vi "FOCUS_V42.vi"(9 "X-pixels":sgl=256.0, 11 "Run":bool) -> (0 "Retrace pixels":sgl, 10 "Pixel Clock (Hz)":sgl)   [LabVIEW 2010] (continued)
                    n2566 = local read "stop 2"() -> (w4780:bool)
                    n2567 = Increment(x=w4762) -> (x+1=w4797:i32)
                    "#" <- w4797
                    n2568 = local read "Overlay Images"() -> (w4801:bool)
                    n2569 = Array Subset "Extract DI0"(array=w4763, index=w4788, length=w4790) -> (w4793:u32[])
                    n2570 = Equal?(x=w4797, y=w4776) -> (x = y?=w4778:bool)
                    n2571 = Split Number(x=w4793) -> (hi(x)=w4752:u16[], lo(x)=w4760:u16[])
                    n2572 = case shown="0, Default" w4759 {
                      tunnel: w4752 -> [w4828 w4833 w4838 w4843 w4848 w4853]
                      tunnel: [w4827 w4832 w4835 w4842 w4847 w4850] -> w4757
                      tunnel: [w4825 w4830 w4837 w4840 w4845 w4852] -> w4756
                      tunnel: w4760 -> [w4826 w4831 w4836 w4841 w4846 w4851]
                      tunnel: [w4824 w4829 w4834 w4839 w4844 w4849] -> w4758
                      frame 0, Default {
                        n2573 = Split Number(x=w4828) -> (hi(x)=w4827:u8[], lo(x)=w4825:u8[])
                        n2574 = Split Number(x=w4826) -> (lo(x)=w4824:u8[])  [unwired: 1 out]
                      }
                      frame 1 {
                        n2575 = Split Number(x=w4833) -> (hi(x)=w4832:u8[], lo(x)=w4829:u8[])
                        n2576 = Split Number(x=w4831) -> (lo(x)=w4830:u8[])  [unwired: 1 out]
                      }
                      frame 2 {
                        n2577 = Split Number(x=w4838) -> (hi(x)=w4834:u8[], lo(x)=w4837:u8[])
                        n2578 = Split Number(x=w4836) -> (lo(x)=w4835:u8[])  [unwired: 1 out]
                      }
                      frame 3 {
                        n2579 = Split Number(x=w4843) -> (hi(x)=w4842:u8[], lo(x)=w4840:u8[])
                        n2580 = Split Number(x=w4841) -> (lo(x)=w4839:u8[])  [unwired: 1 out]
                      }
                      frame 4 {
                        n2581 = Split Number(x=w4848) -> (hi(x)=w4847:u8[], lo(x)=w4844:u8[])
                        n2582 = Split Number(x=w4846) -> (lo(x)=w4845:u8[])  [unwired: 1 out]
                      }
                      frame 5 {
                        n2583 = Split Number(x=w4853) -> (hi(x)=w4849:u8[], lo(x)=w4852:u8[])
                        n2584 = Split Number(x=w4851) -> (lo(x)=w4850:u8[])  [unwired: 1 out]
                      }
                    }
                    n2585 = Set File Position(refnum=w4774, from (0:start)=enum16{"start", "end", "current"}."current" ("pos mode (0:2)"), error in=w4773) -> (refnum out=w4749:refnum<file>, error out=w4748:errorcluster)  [unwired: 1 in]
                    n2586 = Compound Arithmetic op=OR(w4778, w4779, w4780, w4782, w4781, w4783, w4784) -> (w4777:bool)
                    n2587 = Tick Count (ms)() -> (millisecond timer value=w4809:u32)
                    n2588 = case shown="1" w4761 {
                      tunnel: w4757 -> [w4856 w4864]
                      tunnel: [w4856 w4863] -> w4755
                      tunnel: w4762 -> [_ w4859]
                      tunnel: w4756 -> [w4855 w4861]
                      tunnel: [w4855 w4860] -> w4754
                      tunnel: w4758 -> [w4854 w4858]
                      tunnel: [w4854 w4857] -> w4753
                      frame 0, Default {
                      }
                      frame 1 {
                        n2589 = local read "Shift"() -> (w4862:sgl)
                        n2590 = call "testoddevenFOCUS.vi"("Numeric"=w4859) -> ("Boolean"=w4865:bool)
                        n2591 = case shown="True" w4865 {
                          tunnel: w4864 -> [w4868 w4895]
                          tunnel: [w4868 w4897] -> w4863
                          tunnel: w4862 -> [_ w4871]
                          tunnel: w4861 -> [w4867 w4883]
                          tunnel: [w4867 w4882] -> w4860
                          tunnel: w4858 -> [w4866 w4870]
                          tunnel: [w4866 w4869] -> w4857
                          frame False {
                          }
                          frame True {
                            n2592 = Round Toward -Infinity(1:w4871) -> (0:w4887:sgl)
                            n2593 = Round Toward -Infinity(1:w4871) -> (0:w4878:sgl)
                            n2594 = Round Toward -Infinity(1:w4871) -> (0:w4902:sgl)
                            n2595 = To Word Integer(number=w4883) -> (16bit integer=w4893:i16[])
                            n2596 = To Word Integer(number=w4870) -> (16bit integer=w4872:i16[])
                            n2597 = To Word Integer(number=w4895) -> (16bit integer=w4894:i16[])
                            n2598 = Array Subset(array=w4893, index=1) -> (w4886:i16[])  [unwired: 1 in]
                            n2599 = Array Subset(array=w4872, index=1) -> (w4879:i16[])  [unwired: 1 in]
                            n2600 = Array Subset(array=w4894, index=1) -> (w4903:i16[])  [unwired: 1 in]
                            n2601 = Subtract(x=w4871, y=w4887) -> (x-y=w4888:sgl)
                            n2602 = Subtract(x=w4871, y=w4878) -> (x-y=w4877:sgl)
                            n2603 = Subtract(x=w4871, y=w4902) -> (x-y=w4901:sgl)
                            n2604 = Subtract(x=w4893, y=w4886) -> (x-y=w4890:i16[])
                            n2605 = Subtract(x=w4872, y=w4879) -> (x-y=w4875:i16[])
                            n2606 = Subtract(x=w4894, y=w4903) -> (x-y=w4899:i16[])
                            n2607 = Build Array (concatenate)(0 ("index"), w4890) -> (w4891:i32[])
                            n2608 = Build Array (concatenate)(0 ("index"), w4875) -> (w4874:i32[])
                            n2609 = Build Array (concatenate)(0 ("index"), w4899) -> (w4898:i32[])
                            n2610 = Multiply(x=w4888, y=w4891) -> (x*y=w4889:sgl[])
                            n2611 = Multiply(x=w4877, y=w4874) -> (x*y=w4876:sgl[])
                            n2612 = Multiply(x=w4901, y=w4898) -> (x*y=w4900:sgl[])
                            n2613 = Add(x=w4893, y=w4889) -> (x+y=w4884:sgl[])
                            n2614 = To Unsigned Byte Integer(number=w4884) -> (unsigned 8bit integer=w4882:u8[])
                            n2615 = Add(x=w4872, y=w4876) -> (x+y=w4881:sgl[])
                            n2616 = To Unsigned Byte Integer(number=w4881) -> (unsigned 8bit integer=w4869:u8[])
                            n2617 = Add(x=w4894, y=w4900) -> (x+y=w4905:sgl[])
                            n2618 = To Unsigned Byte Integer(number=w4905) -> (unsigned 8bit integer=w4897:u8[])
                          }
                        }
                      }
                    }
                    n2619 = case shown="True" w4801 {
                      tunnel: w4755 -> [w4925 w4928]
                      tunnel: [w4925 w4926] -> w4803
                      tunnel: w4754 -> [w4924 w4927]
                      tunnel: [w4924 _] -> w4802
                      frame False {
                      }
                      frame True {
                        n2620 = To Word Integer(number=w4928) -> (16bit integer=w4933:i16[])
                        n2621 = Subtract(x=w4933, y=w4927) -> (x-y=w4934:i16[])
                        n2622 = Add(x=w4933, y=w4927) -> (x+y=w4938:i16[])
                        n2623 = Increment(x=w4938) -> (x+1=w4929:i16[])
                        n2624 = Divide(x=w4934, y=w4929) -> (x/y=w4930:dbl[])
                        n2625 = Absolute Value(x=w4934) -> (abs(x)=w4936:i16[])
                        n2626 = Multiply(x=w4930, y=u8 2) -> (x*y=w4932:dbl[])
                        n2627 = Round To Nearest(number=w4932) -> (nearest integer value=w4945:dbl[])
                        n2628 = Divide(x=w4936, y=2.0) -> (x/y=w4939:dbl[])
                        n2629 = Divide(x=w4938, y=2.0) -> (x/y=w4940:dbl[])
                        n2630 = Add(x=w4939, y=w4940) -> (x+y=w4942:dbl[])
                        n2631 = Divide(x=w4942, y=5.0) -> (x/y=w4943:dbl[])
                        n2632 = Round To Nearest(number=w4943) -> (nearest integer value=w4944:dbl[])
                        n2633 = Multiply(x=5.0 ("y"), y=w4944) -> (x*y=w4946:dbl[])
                        n2634 = Add(x=w4945, y=w4946) -> (x+y=w4947:dbl[])
                        n2635 = Subtract(x=w4947, y=2.0) -> (x-y=w4950:dbl[])
                        n2636 = To Unsigned Byte Integer(number=w4950) -> (unsigned 8bit integer=w4926:u8[])
                      }
                    }
                    n2637 = Subtract(x=w4762, y=w4790) -> (x-y=w4791:sgl)
                    n2638 = Subtract(x=w4809, y=w4808) -> (x-y=w4810:u32)
                    n2639 = local read "Image Update [ms]"() -> (w4792:u32)
                    n2640 = property class="DAQmx Read"(reference=w4770, error in=w4768) -> (reference out=w4769:refnum<k21>, error out=w4767:errorcluster, "Status:Available Samples Per Channel"=w4766:u32)
                    n2641 = Greater Or Equal?(x=w4810, y=w4792) -> (x >= y?=w4811:bool)
                    n2642 = local write "Scan Backlock"(w4766) -> ()
                    n2643 = case shown="True" w4750 {
                      tunnel: w4755 -> [w4820 w4823]
                      tunnel: w4754 -> [w4817 w4822]
                      tunnel: w4753 -> [w4819 _]
                      tunnel: [w4818 w4821] -> w4751
                      frame True {
                        n2644 = Interleave 1D Arrays(w4817, w4820, w4819) -> (w4818:u8[])
                      }
                      frame False {
                        n2645 = Interleave 1D Arrays(w4823, w4822) -> (w4821:u8[])
                      }
                    }
                    n2646 = Write to Binary File(file (use dialog)=w4749, data=w4751, error in=w4748, 5:FALSE ("prepend array or string size? (T)")) -> (refnum out=w4772:refnum<file>, error out=w4771:errorcluster)  [unwired: 2 in, 1 out]
                    n2647 = local read "X-pixels"() -> (w4812:sgl)
                    n2648 = Subtract(x=w4762, y=w4812) -> (x-y=w4804:sgl)
                    n2649 = Replace Array Subset(array=w4816, new element=w4803, index (col)=w4762) -> (w4814:u8[][])  [unwired: 1 in]
                    n2650 = Replace Array Subset(array=w4815, new element=w4802, index (col)=w4762) -> (w4813:u8[][])  [unwired: 1 in]
                    n2651 = Array Subset(array=w4814, index (col)=w4804, length (col)=w4812) -> (w4806:u8[][])  [unwired: 2 in]
                    n2652 = Array Subset(array=w4813, index (col)=w4804, length (col)=w4812) -> (w4805:u8[][])  [unwired: 2 in]
                    n2653 = case shown="True" w4811 {
                      tunnel: [w4951 w4954] -> w4807
                      tunnel: w4808 -> [w4951 _]
                      tunnel: w4806 -> [_ w4953]
                      tunnel: w4805 -> [_ w4952]
                      frame False {
                      }
                      frame True {
                        n2654 = local write "Image 2"(w4952) -> ()
                        n2655 = local write "Image 1"(w4953) -> ()
                        n2656 = Tick Count (ms)() -> (millisecond timer value=w4954:u32)
                      }
                    }
                  }
                  n2657 = Close File(refnum=w4698, error in=w4699) -> ()  [unwired: 2 out]
                  n2658 = flat-sequence {
                    tunnel: w4731 -> [w4745]
                    tunnel: [w4745] -> w4730
                    frame #0 {
                      n2659 = Tick Count (ms)() -> (millisecond timer value=w4746:u32)
                      n2660 = local write "stop"(w4746) -> ()
                    }
                  }
                }
                frame 3 {
                  w5004 = 0.0 ("X Scale.Range:Minimum")
                  w5017 = 0.0 ("x offset")
                  w5018 = 1.0 ("x offset")
                  w5006 = TRUE ("Visible")
                  # "User-defined line"
                  n2661 = property on="Property Node" class="VI"() -> ("VI Path"=w4972:path)  [unwired: 2 in, 2 out]
                  n2662 = flat-sequence {
                    tunnel: w5011 -> [w5033]
                    tunnel: [w5033] -> w5010
                    frame #0 {
                      n2663 = Tick Count (ms)() -> (millisecond timer value=w5034:u32)
                      n2664 = local write "start"(w5034) -> ()
                    }
                  }
                  n2665 = Greater Or Equal?(x=w4960, y=u16 3) -> (x >= y?=w4958:bool)
                  n2666 = Strip Path(path=w4972) -> (stripped path=w4971:path)  [unwired: 1 out]
                  n2667 = Tick Count (ms)() -> (millisecond timer value=w5024:u32)
                  n2668 = Bundle("x offset"=w5018, "x offset"=w5018, "x offset"=w5017, "x offset"=w5017) -> (w5016:T33)  [unwired: 1 in]
                  n2669 = Build Path(base path=w4971, name or relative path="FreeLine.tmp") -> (appended path=w4970:path)
                  n2670 = Unbundle By Name(w4986) -> ("status"=w4985:bool)
                  n2671 = call <vilib>:"Open_Create_Replace File.vi"("advisory dialog? (display:T)"=FALSE, "function (open:0)"=T8."create or replace", "file path"=w4970) -> ("error out"=w4964:errorcluster, "refnum"=w4966:refnum<file>)  [unwired: 5 in, 2 out]
                  n2672 = Set File Position(refnum=w4966, from (0:start)=enum16{"start", "end", "current"}."start" ("pos mode (rel. to end:1)"), error in=w4964) -> (refnum out=w4957:refnum<file>, error out=w4956:errorcluster)  [unwired: 1 in]
                  n2673 = Write to Binary File(file (use dialog)=w4957, data=w4962, error in=w4956, 5:FALSE ("prepend array or string size? (T)")) -> (refnum out=w4965:refnum<file>, error out=w4963:errorcluster)  [unwired: 2 in, 1 out]
                  n2674 = while {
                    tunnel: [w5054] -> w5025
                    tunnel: [w5055] -> w5009
                    tunnel: w5026 -> [w5100]
                    tunnel: w5010 -> [w5099]
                    shift-right: [w5115] -> w4978
                    shift-left: w5027 -> [w5141]
                    tunnel: w4988 -> [w5097]
                    shift-right: [w5116] -> w4977
                    shift-left: w5027 -> [w5140]
                    shift-right: [w5134] -> _
                    shift-left: w5024 -> [w5135]
                    tunnel: w5022 -> [w5126]
                    tunnel: w5021 -> [w5090]
                    tunnel: [w5125] -> w5020
                    tunnel: [w5124] -> w5019
                    shift-right: [w5121] -> _
                    shift-left: w5016 -> [w5128]
                    tunnel: w5015 -> [w5103]
                    tunnel: w5014 -> [w5091]
                    tunnel: [w5102] -> w5013
                    tunnel: [w5101] -> w5012
                    shift-right: [w5106] -> w4968
                    shift-left: w5002 -> [w5108]
                    tunnel: w4992 -> [w5104]
                    tunnel: w4991 -> [w5082]
                    tunnel: [w5104] -> w4990
                    tunnel: [w5082] -> w4989
                    tunnel: [w5094] -> w4987
                    tunnel: w4985 -> [w5089]
                    shift-right: [w5058] -> w4976
                    shift-left: w4965 -> [w5061]
                    shift-right: [w5059] -> w4975
                    shift-left: w4963 -> [w5060]
                    tunnel: w4961 -> [w5052]
                    tunnel: w4960 -> [w5044]
                    tunnel: w4958 -> [w5038]
                    i -> [w5093]
                    stop <- w5080 stop-if-true
                    # "DIO Read reads one\nline of data at a time"
                    n2675 = Equal To 0?(x=w5093) -> (x = 0?=w5112:bool)
                    n2676 = local read "End experiment"() -> (w5087:bool)
                    n2677 = case shown="True" w5112 {
                      tunnel: w5097 -> [w5207 w5210]
                      tunnel: [w5207 w5209] -> w5049
                      tunnel: w5052 -> [_ w5208]
                      tunnel: [sgl 0.0 w5208] -> w5048
                      frame False {
                      }
                      frame True {
                        n2678 = Add(x=w5210, y=w5208) -> (x+y=w5209:sgl)
                      }
                    }
                    n2679 = call-poly <vilib>:"DAQmx Read (Digital 1D U32 1Chan NSamp).vi"("task/channels in"=w5100, "number of samples per channel"=w5049, "error in"=w5099) -> ("task out"=w5057:refnum<k21>, "data"=w5051:u32[], "error out"=w5056:errorcluster)  [unwired: 10 in]
                    n2680 = Increment(x=w5093) -> (x+1=w5105:i32)
                    "#" <- w5105
                    n2681 = call-poly <vilib>:"DAQmx Read (Analog 2D DBL NChan NSamp).vi"("task/channels in"=w5103, "number of samples per channel"=w5049, "error in"=w5091) -> ("task out"=w5102:refnum<k21>, "data"=w5047:dbl[][], "error out"=w5101:errorcluster)  [unwired: 10 in]
                    n2682 = Unbundle By Name(w5091) -> ("status"=w5081:bool)
                    n2683 = local read "stop 2"() -> (w5088:bool)
                    n2684 = local read "Overlay Images"() -> (w5109:bool)
                    n2685 = Array Subset(array=w5047, index (col)=w5048) -> (w5046:dbl[][])  [unwired: 3 in]
                    n2686 = Unbundle By Name(w5090) -> ("status"=w5083:bool)
                    n2687 = Equal?(x=w5105, y="Y-lines FreeLine") -> (x = y?=w5086:bool)
                    n2688 = Transpose 2D Array(2D array=w5046) -> (transposed array=w5098:dbl[][])
                    n2689 = Unbundle By Name(w5056) -> ("status"=w5084:bool)
                    n2690 = Array Subset "Extract DI0"(array=w5051, index=w5048) -> (w5050:u32[])  [unwired: 1 in]
                    n2691 = Unbundle By Name(w5082) -> ("status"=w5085:bool)
                    n2692 = Split Number(x=w5050) -> (hi(x)=w5040:u16[], lo(x)=w5045:u16[])
                    n2693 = Build Array (concatenate)(w5108, w5098) -> (w5107:dbl[][])
                    n2694 = Index Array(array=w5098, index (col)=0 ("disabled index (col)")) -> (element=w5118:dbl[])  [unwired: 1 in]
                    n2695 = Bundle("x offset"="x offset", "x scale"="x scale", "y offset"="y offset", "y scale"="y scale") -> (w5121:T34)  [unwired: 1 in]
                    n2696 = Array Subset(array=w5107, index (row)=w5097) -> (w5106:dbl[][])  [unwired: 3 in]
                    n2697 = Index Array(array=w5098, index (col)=1 ("disabled index (col)")) -> (element=w5117:dbl[])  [unwired: 1 in]
                    n2698 = Tick Count (ms)() -> (millisecond timer value=w5136:u32)
                    n2699 = Not Equal?(x=w5128, y=w5121) -> (x != y?=w5127:bool)
                    n2700 = Compound Arithmetic op=OR(w5081, w5083, w5084, w5085, w5086, w5087, w5088, w5089) -> (w5080:bool)
                    n2701 = case shown="True" w5127 {
                      tunnel: w5126 -> [w5212 w5217]
                      tunnel: w5090 -> [w5211 w5214]
                      tunnel: [w5212 w5215] -> w5125
                      tunnel: [w5211 w5213] -> w5124
                      tunnel: w5121 -> [_ w5219]
                      frame False {
                      }
                      frame True {
                        n2702 = local read "ScanLineFreeLine"() -> (w5218:sgl[][])
                        n2703 = call "ScaleudlFOCUS.vi"("Cluster"=w5219, "ScanLineUDL"=w5218) -> ("ScanLineUDLnew"=w5216:dbl[][])
                        n2704 = call-poly <vilib>:"DAQmx Write (Analog 2D DBL NChan NSamp).vi"("task/channels in"=w5217, "data"=w5216, "error in"=w5214) -> ("task out"=w5215:refnum<k21>, "error out"=w5213:errorcluster)  [unwired: 10 in, 1 out]
                      }
                    }
                    n2705 = case shown="0, Default" w5044 {
                      tunnel: w5040 -> [w5153 w5158 w5163 w5168 w5173 w5178]
                      tunnel: [w5152 w5157 w5160 w5167 w5172 w5175] -> w5041
                      tunnel: [w5150 w5155 w5162 w5165 w5170 w5177] -> w5042
                      tunnel: w5045 -> [w5151 w5156 w5161 w5166 w5171 w5176]
                      tunnel: [w5149 w5154 w5159 w5164 w5169 w5174] -> w5043
                      frame 0, Default {
                        n2706 = Split Number(x=w5153) -> (hi(x)=w5152:u8[], lo(x)=w5150:u8[])
                        n2707 = Split Number(x=w5151) -> (lo(x)=w5149:u8[])  [unwired: 1 out]
                      }
                      frame 1 {
                        n2708 = Split Number(x=w5158) -> (hi(x)=w5157:u8[], lo(x)=w5154:u8[])
                        n2709 = Split Number(x=w5156) -> (lo(x)=w5155:u8[])  [unwired: 1 out]
                      }
                      frame 2 {
                        n2710 = Split Number(x=w5163) -> (hi(x)=w5159:u8[], lo(x)=w5162:u8[])
                        n2711 = Split Number(x=w5161) -> (lo(x)=w5160:u8[])  [unwired: 1 out]
                      }
                      frame 3 {
                        n2712 = Split Number(x=w5168) -> (hi(x)=w5167:u8[], lo(x)=w5165:u8[])
                        n2713 = Split Number(x=w5166) -> (lo(x)=w5164:u8[])  [unwired: 1 out]
                      }
                      frame 4 {
                        n2714 = Split Number(x=w5173) -> (hi(x)=w5172:u8[], lo(x)=w5169:u8[])
                        n2715 = Split Number(x=w5171) -> (lo(x)=w5170:u8[])  [unwired: 1 out]
                      }
                      frame 5 {
                        n2716 = Split Number(x=w5178) -> (hi(x)=w5174:u8[], lo(x)=w5177:u8[])
                        n2717 = Split Number(x=w5176) -> (lo(x)=w5175:u8[])  [unwired: 1 out]
                      }
                    }
                    n2718 = case shown="True" w5109 {
                      tunnel: w5041 -> [w5180 w5183]
                      tunnel: [w5180 w5181] -> w5111
                      tunnel: w5042 -> [w5179 w5182]
                      tunnel: [w5179 _] -> w5110
                      frame False {
                      }
                      frame True {
                        n2719 = To Word Integer(number=w5183) -> (16bit integer=w5188:i16[])
                        n2720 = Subtract(x=w5188, y=w5182) -> (x-y=w5189:i16[])
                        n2721 = Add(x=w5188, y=w5182) -> (x+y=w5193:i16[])
                        n2722 = Increment(x=w5193) -> (x+1=w5184:i16[])
                        n2723 = Divide(x=w5189, y=w5184) -> (x/y=w5185:dbl[])
                        n2724 = Absolute Value(x=w5189) -> (abs(x)=w5191:i16[])
                        n2725 = Multiply(x=w5185, y=u8 2) -> (x*y=w5187:dbl[])
                        n2726 = Round To Nearest(number=w5187) -> (nearest integer value=w5200:dbl[])
                        n2727 = Divide(x=w5191, y=2.0) -> (x/y=w5194:dbl[])
                        n2728 = Divide(x=w5193, y=2.0) -> (x/y=w5195:dbl[])
                        n2729 = Add(x=w5194, y=w5195) -> (x+y=w5197:dbl[])
                        n2730 = Divide(x=w5197, y=5.0) -> (x/y=w5198:dbl[])
                        n2731 = Round To Nearest(number=w5198) -> (nearest integer value=w5199:dbl[])
                        n2732 = Multiply(x=5.0 ("y"), y=w5199) -> (x*y=w5201:dbl[])
                        n2733 = Add(x=w5200, y=w5201) -> (x+y=w5202:dbl[])
                        n2734 = Subtract(x=w5202, y=2.0) -> (x-y=w5205:dbl[])
                        n2735 = To Unsigned Byte Integer(number=w5205) -> (unsigned 8bit integer=w5181:u8[])
                      }
                    }
                    n2736 = Subtract(x=w5136, y=w5135) -> (x-y=w5137:u32)
                    n2737 = local read "Image Update [ms]"() -> (w5096:u32)
                    n2738 = property class="DAQmx Read"(reference=w5057, error in=w5056) -> (reference out=w5054:refnum<k21>, error out=w5055:errorcluster, "Status:Available Samples Per Channel"=w5053:u32)
                    n2739 = Multiply(x="x scale", y=w5118) -> (x*y=w5132:dbl[])
                    n2740 = Greater Or Equal?(x=w5137, y=w5096) -> (x >= y?=w5138:bool)
                    n2741 = Multiply(x=w5117, y="y scale") -> (x*y=w5131:dbl[])
                    n2742 = case shown="True" w5038 {
                      tunnel: w5041 -> [w5145 w5148]
                      tunnel: w5042 -> [w5142 w5147]
                      tunnel: w5043 -> [w5144 _]
                      tunnel: [w5143 w5146] -> w5039
                      frame True {
                        n2743 = Interleave 1D Arrays(w5142, w5145, w5144) -> (w5143:u8[])
                      }
                      frame False {
                        n2744 = Interleave 1D Arrays(w5148, w5147) -> (w5146:u8[])
                      }
                    }
                    n2745 = Add(x="x offset", y=w5132) -> (x+y=w5064:dbl[])
                    n2746 = Add(x=w5131, y="y offset") -> (x+y=w5066:dbl[])
                    n2747 = local write "Scan Backlock"(w5053) -> ()
                    n2748 = local read "y jog"() -> (w5067:sgl)
                    n2749 = local read "x jog"() -> (w5068:sgl)
                    n2750 = Subtract(x=w5066, y=w5067) -> (x-y=w5065:dbl[])
                    n2751 = Subtract(x=w5064, y=w5068) -> (x-y=w5063:dbl[])
                    n2752 = local read "Zoom"() -> (w5069:sgl)
                    n2753 = local read "X-pixels FreeLine"() -> (w5095:sgl)
                    n2754 = Replace Array Subset(array=w5141, new element=w5111, index (col)=w5093) -> (w5115:u8[][])  [unwired: 1 in]
                    n2755 = Replace Array Subset(array=w5140, new element=w5110, index (col)=w5093) -> (w5116:u8[][])  [unwired: 1 in]
                    n2756 = Multiply(x=w5065, y=w5069) -> (x*y=w5071:dbl[])
                    n2757 = Multiply(x=w5063, y=w5069) -> (x*y=w5070:dbl[])
                    n2758 = Subtract(x=w5093, y=w5095) -> (x-y=w5139:sgl)
                    n2759 = Set File Position(refnum=w5061, from (0:start)=enum16{"start", "end", "current"}."current" ("pos mode (0:2)"), error in=w5060) -> (refnum out=w5037:refnum<file>, error out=w5036:errorcluster)  [unwired: 1 in]
                    n2760 = Write to Binary File(file (use dialog)=w5037, data=w5039, error in=w5036, 5:FALSE ("prepend array or string size? (T)")) -> (refnum out=w5058:refnum<file>, error out=w5059:errorcluster)  [unwired: 2 in, 1 out]
                    n2761 = Array Subset(array=w5115, index (col)=w5139, length (col)=w5095) -> (w5114:u8[][])  [unwired: 2 in]
                    n2762 = Multiply(x=sgl -2.7 ("X Factor"), y=w5071) -> (x*y=w5077:dbl[])
                    n2763 = Multiply(x=sgl -2.7 ("X Factor"), y=w5070) -> (x*y=w5073:dbl[])
                    n2764 = Subtract(x=w5093, y=w5095) -> (x-y=w5094:sgl)
                    n2765 = Array Subset(array=w5116, index (col)=w5139, length (col)=w5095) -> (w5113:u8[][])  [unwired: 2 in]
                    n2766 = Add(x=sgl -0.005 ("X Offset"), y=w5077) -> (x+y=w5076:dbl[])
                    n2767 = Add(x=sgl -0.025 ("X Offset"), y=w5073) -> (x+y=w5072:dbl[])
                    n2768 = Bundle(w5072, w5076) -> (w5133:cluster{dbl[], dbl[]})  [unwired: 1 in]
                    n2769 = case shown="True" w5138 {
                      tunnel: [w5220 w5224] -> w5134
                      tunnel: w5135 -> [w5220 _]
                      tunnel: w5133 -> [_ w5223]
                      tunnel: w5114 -> [_ w5222]
                      tunnel: w5113 -> [_ w5221]
                      frame False {
                      }
                      frame True {
                        n2770 = local write "XY Graph 3"(w5223) -> ()
                        n2771 = local write "XY Graph 4"(w5223) -> ()
                        n2772 = local write "Image 4"(w5221) -> ()
                        n2773 = local write "Image 3"(w5222) -> ()
                        n2774 = Tick Count (ms)() -> (millisecond timer value=w5224:u32)
                      }
                    }
                  }
                  n2775 = local read "X-pixels FreeLine"() -> (w5007:sgl)
                  n2776 = property on="Image 2" class="IntGraph (strict)"() -> ("Color Table"=w5005:u32[])  [unwired: 2 in, 2 out]
                  n2777 = Decrement(x=w5007) -> (x-1=w5003:sgl)
                  n2778 = property on="Image 3" class="IntGraph (strict)"("X Scale.Range:Minimum"=w5004, "X Scale.Range:Maximum"=w5003, "Y Scale.Range:Minimum"=w5004, "Y Scale.Range:Maximum"=w5003, "Visible"=w5006, "Color Table"=w5005) -> ()  [unwired: 2 in, 2 out]
                  n2779 = property on="Image 4" class="IntGraph (strict)"("X Scale.Range:Minimum"=w5004, "X Scale.Range:Maximum"=w5003, "Y Scale.Range:Minimum"=w5004, "Y Scale.Range:Maximum"=w5003, "Visible"=w5006, "Color Table"=w5005) -> ()  [unwired: 2 in, 2 out]
                  n2780 = property on="Histogram1" class="XYGraph (strict)"("X Scale.Range:Minimum"=w5004, "X Scale.Range:Maximum"=w5003) -> ()  [unwired: 2 in, 2 out]
                  n2781 = property on="Histogram2" class="XYGraph (strict)"("X Scale.Range:Minimum"=w5004, "X Scale.Range:Maximum"=w5003) -> ()  [unwired: 2 in, 2 out]
                  n2782 = Close File(refnum=w4976, error in=w4975) -> ()  [unwired: 2 out]
                  n2783 = Array Subset(array=w4968, index (col)=0 ("index"), length (col)=3 ("length")) -> (w4993:dbl[][])  [unwired: 2 in]
                  n2784 = Index Array(array=w4993, index (col)=0 ("disabled index (col)")) -> (element=w5000:dbl[])  [unwired: 1 in]
                  n2785 = Array Size(array=w5000) -> (size(s)=w4999:i32)
                  n2786 = Multiply(x=w4999, y=3) -> (x*y=w4997:i32)
                  n2787 = Reshape Array(w4993, w4997) -> (→"Positions":dbl[])
                  n2788 = flat-sequence {
                    tunnel: [w5031] -> w5008
                    tunnel: w5009 -> [w5031]
                    frame #0 {
                      n2789 = Tick Count (ms)() -> (millisecond timer value=w5032:u32)
                      n2790 = local write "stop"(w5032) -> ()
                    }
                  }
                }
                frame 4 {
                  # "Iinner while loop runs for n loops, where n = number of averages.\nAll data acquired in this loop enters the average.\nThe z-step is activated each time this loop completes..\nThe outer while loop iterates m times, where m is total number of frames.\nControls are reset after the outer while loop completes.\nThe shutter is closed before and opened after each z-step."
                  # "Frame scan piezo"
                  n2791 = local read "z-step (um)"() -> (w5230:sgl)
                  n2792 = flat-sequence {
                    tunnel: w5287 -> [w5304]
                    tunnel: [w5304] -> w5286
                    frame #0 {
                      n2793 = Tick Count (ms)() -> (millisecond timer value=w5305:u32)
                      n2794 = local write "start"(w5305) -> ()
                    }
                  }
                  n2795 = local read "Number of frames"() -> (w5288:sgl)
                  n2796 = Unbundle By Name(w5257) -> ("status"=w5256:bool)
                  n2797 = local read "z-step (um)"() -> (w5295:sgl)
                  n2798 = property on="Property Node" class="VI"() -> ("VI Path"=w5244:path)  [unwired: 2 in, 2 out]
                  n2799 = Initialize Array(u8 0 ("element"), w5271, w5272) -> (w5284:u8[][])
                  n2800 = Equal To 0?(x=w5230) -> (x = 0?=w5229:bool)
                  n2801 = Initialize Array(0.0 ("element"), 0 ("dimension size")) -> (w5294:dbl[])
                  n2802 = Strip Path(path=w5244) -> (stripped path=w5243:path)  [unwired: 1 out]
                  n2803 = while {
                    tunnel: w5295 -> [w5316]
                    shift-right: [w5314] -> w5290
                    shift-left: w5294 -> [w5315]
                    tunnel: w5288 -> [w5308]
                    i -> [w5307]
                    stop <- w5309 stop-if-true
                    n2804 = Multiply(x=w5316, y=w5307) -> (x*y=w5312:sgl)
                    n2805 = Increment(x=w5307) -> (x+1=w5306:i32)
                    n2806 = Build Array (concatenate)(w5315, w5312) -> (w5314:dbl[])
                    n2807 = Greater Or Equal?(x=w5312, y=400.0) -> (x >= y?=w5310:bool)
                    n2808 = Greater Or Equal?(x=w5306, y=w5308) -> (x >= y?=w5311:bool)
                    n2809 = Or(x=w5310, y=w5311) -> (x .or. y?=w5309:bool)
                  }
                  n2810 = Build Path(base path=w5243, name or relative path="Stack.tmp") -> (appended path=w5242:path)
                  n2811 = call <vilib>:"Open_Create_Replace File.vi"("advisory dialog? (display:T)"=FALSE, "function (open:0)"=T8."create or replace", "file path"=w5242) -> ("error out"=w5235:errorcluster, "refnum"=w5237:refnum<file>)  [unwired: 5 in, 2 out]
                  n2812 = Divide(x=w5290, y=40.0) -> (x/y=w5268:dbl[])
                  n2813 = Set File Position(refnum=w5237, from (0:start)=enum16{"start", "end", "current"}."start" ("pos mode (rel. to end:1)"), error in=w5235) -> (refnum out=w5227:refnum<file>, error out=w5226:errorcluster)  [unwired: 1 in]
                  n2814 = Write to Binary File(file (use dialog)=w5227, data=w5233, error in=w5226, 5:FALSE ("prepend array or string size? (T)")) -> (refnum out=w5236:refnum<file>, error out=w5234:errorcluster)  [unwired: 2 in, 1 out]
                  n2815 = Array Subset(array=w5268, index=1) -> (w5267:dbl[])  [unwired: 1 in]
                  n2816 = local read "IntensityAutomatic"() -> (w5252:bool)
                  n2817 = local read "Intensity"() -> (w5254:sgl)
                  n2818 = while {
                    tunnel: [w5392] -> w5266
                    tunnel: [w5391] -> w5265
                    tunnel: w5300 -> [w5390]
                    tunnel: w5286 -> [w5349]
                    tunnel: w5299 -> [w5325]
                    tunnel: w5289 -> [w5389]
                    tunnel: w5267 -> [w5360] mode=indexing
                    tunnel: w5268 -> [w5388]
                    shift-right: [w5386] -> w5250
                    shift-left: w5284 -> [w5387]
                    shift-right: [w5384] -> w5251
                    shift-left: w5284 -> [w5385]
                    tunnel: w5280 -> [w5383]
                    tunnel: w5279 -> [w5352]
                    tunnel: [w5382] -> w5277
                    tunnel: [w5381] -> w5278
                    tunnel: w5276 -> [w5366]
                    tunnel: w5275 -> [w5365]
                    tunnel: [w5371] -> w5274
                    tunnel: [w5370] -> w5273
                    tunnel: [w5356] -> w5270
                    tunnel: w5260 -> [w5364]
                    tunnel: [w5357] -> w5261
                    tunnel: w5254 -> [w5359]
                    tunnel: w5259 -> [w5355]
                    tunnel: [w5353] -> w5258
                    tunnel: w5256 -> [w5347]
                    tunnel: [w5341] -> w5253
                    tunnel: w5252 -> [w5340]
                    shift-right: [w5336] -> w5240
                    shift-left: w5236 -> [w5338]
                    shift-right: [w5335] -> w5239
                    shift-left: w5234 -> [w5337]
                    tunnel: w5232 -> [w5331]
                    tunnel: w5231 -> [w5322]
                    tunnel: w5229 -> [w5328]
                    tunnel: w5228 -> [w5321]
                    i -> [w5353]
                    stop <- w5327 stop-if-true
                    n2819 = Equal To 0?(x=w5353) -> (x = 0?=w5329:bool)
                    n2820 = Or(x=w5329, y=w5328) -> (x .or. y?=w5330:bool)
                    n2821 = case shown="False" w5330 {
                      tunnel: w5366 -> [w5468 w5477]
                      tunnel: [w5461 w5477] -> w5361
                      tunnel: w5365 -> [w5467 w5478]
                      tunnel: [w5460 w5478] -> w5351
                      tunnel: w5355 -> [w5465 w5475]
                      tunnel: w5364 -> [w5464 w5476]
                      tunnel: [w5459 w5476] -> w5350
                      tunnel: [w5458 w5475] -> w5363
                      frame False {
                        w5466 = TRUE ("data")
                        n2822 = local write "Shutter open"(w5466) -> ()
                        n2823 = call-poly <vilib>:"DAQmx Write (Digital Bool 1Line 1Point).vi"("task/channels in"=w5468, "data"=w5466, "error in"=w5467) -> ("task out"=w5463:refnum<k21>, "error out"=w5462:errorcluster)  [unwired: 10 in, 1 out]
                        n2824 = flat-sequence {
                          tunnel: w5465 -> [w5474]
                          tunnel: w5464 -> [w5473]
                          tunnel: w5463 -> [w5472]
                          tunnel: [w5472] -> w5461
                          tunnel: [w5471] -> w5460
                          tunnel: w5462 -> [w5471]
                          tunnel: [w5470] -> w5459
                          tunnel: [w5469] -> w5458
                          frame #0 {
                            n2825 = call <vilib>:"DAQmx Start Task.vi"("task/channels in"=w5474, "error in"=w5473) -> ("task out"=w5469:refnum<k21>, "error out"=w5470:errorcluster)  [unwired: 12 in]
                          }
                        }
                      }
                      frame True {
                      }
                    }
                    n2826 = Greater Or Equal?(x=w5321, y=u16 3) -> (x >= y?=w5320:bool)
                    n2827 = local read "Number of frames"() -> (w5354:sgl)
                    n2828 = Tick Count (ms)() -> (millisecond timer value=w5373:u32)
                    n2829 = Array Size(array=w5388) -> (size(s)=w5376:i32)
                    n2830 = Unbundle By Name(w5352) -> ("status"=w5348:bool)
                    n2831 = Increment(x=w5353) -> (x+1=w5372:i32)
                    n2832 = Equal?(x=w5354, y=w5372) -> (x = y?=w5374:bool)
                    n2833 = Equal?(x=w5372, y=w5376) -> (x = y?=w5375:bool)
                    n2834 = Compound Arithmetic op=OR(w5348, w5347) -> (w5345:bool)
                    n2835 = while {
                      tunnel: [w5509] -> w5392
                      tunnel: [w5511] -> w5391
                      tunnel: w5390 -> [w5558]
                      tunnel: w5349 -> [w5557]
                      shift-right: [w5544] -> w5334
                      shift-left: w5325 -> [w5545]
                      tunnel: w5389 -> [w5528]
                      shift-right: [w5540] -> w5333
                      shift-left: w5325 -> [w5543]
                      tunnel: [w5516] -> w5344
                      tunnel: [w5517] -> w5343
                      shift-right: [w5561] -> _
                      shift-left: w5373 -> [w5562]
                      tunnel: [w5532] -> w5369
                      tunnel: w5361 -> [w5532]
                      tunnel: [w5522] -> w5367
                      tunnel: w5351 -> [w5522]
                      tunnel: [w5531] -> w5358
                      tunnel: w5363 -> [w5531]
                      tunnel: [w5523] -> w5362
                      tunnel: w5350 -> [w5523]
                      tunnel: w5345 -> [w5515]
                      tunnel: [w5513] -> w5342
                      tunnel: w5331 -> [w5507]
                      tunnel: w5322 -> [w5496]
                      tunnel: w5329 -> [w5503]
                      shift-right: [w5482] -> w5324
                      shift-left: w5325 -> [w5484]
                      tunnel: w5321 -> [w5481]
                      i -> [w5495]
                      stop <- w5514 stop-if-true
                      # "DIO Read reads one\nline of data at a time"
                      n2836 = local read "z-step (um)"() -> (w5505:sgl)
                      n2837 = local read "Scan Cut-Off (either end)"() -> (w5559:sgl)
                      n2838 = local read "End experiment"() -> (w5517:bool)
                      n2839 = Equal To 0?(x=w5495) -> (x = 0?=w5504:bool)
                      n2840 = Equal To 0?(x=w5505) -> (x = 0?=w5506:bool)
                      n2841 = local read "Overlay Images"() -> (w5560:bool)
                      n2842 = Unbundle By Name(w5523) -> ("status"=w5520:bool)
                      n2843 = Unbundle By Name(w5522) -> ("status"=w5519:bool)
                      n2844 = local read "X-pixels"() -> (w5556:sgl)
                      n2845 = local read "Cusp Delay"() -> (w5526:sgl)
                      n2846 = local read "stop 2"() -> (w5516:bool)
                      n2847 = case shown="True" w5506 {
                        tunnel: w5503 -> [_ w5650]
                        tunnel: w5504 -> [w5647 w5649]
                        tunnel: [w5647 w5648] -> w5502
                        frame False {
                        }
                        frame True {
                          n2848 = And(x=w5649, y=w5650) -> (x .and. y?=w5648:bool)
                        }
                      }
                      n2849 = case shown="False" w5502 {
                        tunnel: w5528 -> [w5667 w5672]
                        tunnel: [w5667 w5671] -> w5527
                        tunnel: w5559 -> [w5666 w5670]
                        tunnel: [w5666 w5669] -> w5524
                        tunnel: w5507 -> [_ w5668]
                        frame False {
                        }
                        frame True {
                          n2850 = Add(x=w5672, y=w5668) -> (x+y=w5671:sgl)
                          n2851 = Add(x=w5670, y=w5668) -> (x+y=w5669:sgl)
                        }
                      }
                      n2852 = call-poly <vilib>:"DAQmx Read (Digital 1D U32 1Chan NSamp).vi"("task/channels in"=w5558, "number of samples per channel"=w5527, "error in"=w5557) -> ("task out"=w5510:refnum<k21>, "data"=w5500:u32[], "error out"=w5512:errorcluster)  [unwired: 10 in]
                      n2853 = case shown="1" w5496 {
                        tunnel: w5495 -> [_ w5656]
                        tunnel: w5500 -> [w5651 w5654]
                        tunnel: [w5651 w5653] -> w5499
                        frame 0, Default {
                        }
                        frame 1 {
                          n2854 = local read "Shift"() -> (w5652:sgl)
                          n2855 = call "testoddevenFOCUS.vi"("Numeric"=w5656) -> ("Boolean"=w5655:bool)
                          n2856 = case shown="True" w5655 {
                            tunnel: w5654 -> [w5658 w5661]
                            tunnel: [w5657 w5659] -> w5653
                            tunnel: w5652 -> [_ w5660]
                            frame False {
                              n2857 = Reverse 1D Array(array=w5658) -> (reversed array=w5657:u32[])
                            }
                            frame True {
                              n2858 = Rotate 1D Array(1:w5661, 2:w5660) -> (0:w5659:u32[])
                            }
                          }
                        }
                      }
                      n2859 = Add(x=w5526, y=w5524) -> (x+y=w5525:sgl)
                      n2860 = Array Subset "Extract DI0"(array=w5499, index=w5525, length=w5556) -> (w5501:u32[])
                      n2861 = Split Number(x=w5501) -> (hi(x)=w5494:u16[], lo(x)=w5493:u16[])
                      n2862 = case shown="0, Default" w5481 {
                        tunnel: w5494 -> [w5569 w5574 w5579 w5584 w5589 w5594]
                        tunnel: [w5568 w5573 w5576 w5583 w5588 w5591] -> w5492
                        tunnel: [w5566 w5571 w5578 w5581 w5586 w5593] -> w5491
                        tunnel: w5493 -> [w5567 w5572 w5577 w5582 w5587 w5592]
                        tunnel: [w5565 w5570 w5575 w5580 w5585 w5590] -> w5490
                        frame 0, Default {
                          n2863 = Split Number(x=w5569) -> (hi(x)=w5568:u8[], lo(x)=w5566:u8[])
                          n2864 = Split Number(x=w5567) -> (lo(x)=w5565:u8[])  [unwired: 1 out]
                        }
                        frame 1 {
                          n2865 = Split Number(x=w5574) -> (hi(x)=w5573:u8[], lo(x)=w5570:u8[])
                          n2866 = Split Number(x=w5572) -> (lo(x)=w5571:u8[])  [unwired: 1 out]
                        }
                        frame 2 {
                          n2867 = Split Number(x=w5579) -> (hi(x)=w5575:u8[], lo(x)=w5578:u8[])
                          n2868 = Split Number(x=w5577) -> (lo(x)=w5576:u8[])  [unwired: 1 out]
                        }
                        frame 3 {
                          n2869 = Split Number(x=w5584) -> (hi(x)=w5583:u8[], lo(x)=w5581:u8[])
                          n2870 = Split Number(x=w5582) -> (lo(x)=w5580:u8[])  [unwired: 1 out]
                        }
                        frame 4 {
                          n2871 = Split Number(x=w5589) -> (hi(x)=w5588:u8[], lo(x)=w5585:u8[])
                          n2872 = Split Number(x=w5587) -> (lo(x)=w5586:u8[])  [unwired: 1 out]
                        }
                        frame 5 {
                          n2873 = Split Number(x=w5594) -> (hi(x)=w5590:u8[], lo(x)=w5593:u8[])
                          n2874 = Split Number(x=w5592) -> (lo(x)=w5591:u8[])  [unwired: 1 out]
                        }
                      }
                      n2875 = Unbundle By Name(w5512) -> ("status"=w5521:bool)
                      n2876 = case shown="1" w5496 {
                        tunnel: w5492 -> [w5597 w5604]
                        tunnel: [w5597 w5603] -> w5498
                        tunnel: w5495 -> [_ w5606]
                        tunnel: w5491 -> [w5596 w5601]
                        tunnel: [w5596 w5600] -> w5497
                        tunnel: w5490 -> [w5595 w5599]
                        tunnel: [w5595 w5598] -> w5479
                        frame 0, Default {
                        }
                        frame 1 {
                          n2877 = local read "Shift"() -> (w5602:sgl)
                          n2878 = call "testoddevenFOCUS.vi"("Numeric"=w5606) -> ("Boolean"=w5605:bool)
                          n2879 = case shown="True" w5605 {
                            tunnel: w5604 -> [w5609 w5636]
                            tunnel: [w5609 w5638] -> w5603
                            tunnel: w5602 -> [_ w5612]
                            tunnel: w5601 -> [w5608 w5624]
                            tunnel: [w5608 w5623] -> w5600
                            tunnel: w5599 -> [w5607 w5611]
                            tunnel: [w5607 w5610] -> w5598
                            frame False {
                            }
                            frame True {
                              n2880 = Round Toward -Infinity(1:w5612) -> (0:w5628:sgl)
                              n2881 = Round Toward -Infinity(1:w5612) -> (0:w5643:sgl)
                              n2882 = Round Toward -Infinity(1:w5612) -> (0:w5619:sgl)
                              n2883 = To Word Integer(number=w5624) -> (16bit integer=w5634:i16[])
                              n2884 = To Word Integer(number=w5636) -> (16bit integer=w5635:i16[])
                              n2885 = To Word Integer(number=w5611) -> (16bit integer=w5613:i16[])
                              n2886 = Array Subset(array=w5634, index=1) -> (w5627:i16[])  [unwired: 1 in]
                              n2887 = Array Subset(array=w5635, index=1) -> (w5644:i16[])  [unwired: 1 in]
                              n2888 = Array Subset(array=w5613, index=1) -> (w5620:i16[])  [unwired: 1 in]
                              n2889 = Subtract(x=w5612, y=w5628) -> (x-y=w5629:sgl)
                              n2890 = Subtract(x=w5612, y=w5643) -> (x-y=w5642:sgl)
                              n2891 = Subtract(x=w5612, y=w5619) -> (x-y=w5618:sgl)
                              n2892 = Subtract(x=w5634, y=w5627) -> (x-y=w5631:i16[])
                              n2893 = Subtract(x=w5635, y=w5644) -> (x-y=w5640:i16[])
                              n2894 = Subtract(x=w5613, y=w5620) -> (x-y=w5616:i16[])
                              n2895 = Build Array (concatenate)(0 ("index"), w5631) -> (w5632:i32[])
                              n2896 = Build Array (concatenate)(0 ("index"), w5640) -> (w5639:i32[])
                              n2897 = Build Array (concatenate)(0 ("index"), w5616) -> (w5615:i32[])
                              n2898 = Multiply(x=w5629, y=w5632) -> (x*y=w5630:sgl[])
                              n2899 = Multiply(x=w5642, y=w5639) -> (x*y=w5641:sgl[])
                              n2900 = Multiply(x=w5618, y=w5615) -> (x*y=w5617:sgl[])
                              n2901 = Add(x=w5634, y=w5630) -> (x+y=w5625:sgl[])
                              n2902 = To Unsigned Byte Integer(number=w5625) -> (unsigned 8bit integer=w5623:u8[])
                              n2903 = Add(x=w5635, y=w5641) -> (x+y=w5646:sgl[])
                              n2904 = To Unsigned Byte Integer(number=w5646) -> (unsigned 8bit integer=w5638:u8[])
                              n2905 = Add(x=w5613, y=w5617) -> (x+y=w5622:sgl[])
                              n2906 = To Unsigned Byte Integer(number=w5622) -> (unsigned 8bit integer=w5610:u8[])
                            }
                          }
                        }
                      }
                      n2907 = case shown="True" w5560 {
                        tunnel: w5498 -> [w5674 w5677]
                        tunnel: [w5674 w5675] -> w5542
                        tunnel: w5497 -> [w5673 w5676]
                        tunnel: [w5673 _] -> w5541
                        frame False {
                        }
                        frame True {
                          n2908 = To Word Integer(number=w5677) -> (16bit integer=w5682:i16[])
                          n2909 = Subtract(x=w5682, y=w5676) -> (x-y=w5683:i16[])
                          n2910 = Add(x=w5682, y=w5676) -> (x+y=w5687:i16[])
                          n2911 = Increment(x=w5687) -> (x+1=w5678:i16[])
                          n2912 = Divide(x=w5683, y=w5678) -> (x/y=w5679:dbl[])
                          n2913 = Absolute Value(x=w5683) -> (abs(x)=w5685:i16[])
                          n2914 = Multiply(x=w5679, y=u8 2) -> (x*y=w5681:dbl[])
                          n2915 = Round To Nearest(number=w5681) -> (nearest integer value=w5694:dbl[])
                          n2916 = Divide(x=w5685, y=2.0) -> (x/y=w5688:dbl[])
                          n2917 = Divide(x=w5687, y=2.0) -> (x/y=w5689:dbl[])
                          n2918 = Add(x=w5688, y=w5689) -> (x+y=w5691:dbl[])
                          n2919 = Divide(x=w5691, y=5.0) -> (x/y=w5692:dbl[])
                          n2920 = Round To Nearest(number=w5692) -> (nearest integer value=w5693:dbl[])
                          n2921 = Multiply(x=5.0 ("y"), y=w5693) -> (x*y=w5695:dbl[])
                          n2922 = Add(x=w5694, y=w5695) -> (x+y=w5696:dbl[])
                          n2923 = Subtract(x=w5696, y=2.0) -> (x-y=w5699:dbl[])
                          n2924 = To Unsigned Byte Integer(number=w5699) -> (unsigned 8bit integer=w5675:u8[])
                        }
                      }
                      n2925 = Compound Arithmetic op=OR(w5521, w5520, w5519) -> (w5513:bool)
                      n2926 = property class="DAQmx Read"(reference=w5510, error in=w5512) -> (reference out=w5509:refnum<k21>, error out=w5511:errorcluster, "Status:Available Samples Per Channel"=w5508:u32)
                      n2927 = local read "total y pixels"() -> (w5536:sgl)
                      n2928 = local read "Averaging"() -> (w5539:u16)
                      n2929 = local write "Scan Backlock"(w5508) -> ()
                      n2930 = Multiply(x=w5536, y=w5539) -> (x*y=w5563:sgl)
                      n2931 = Increment(x=w5495) -> (x+1=w5537:i32)
                      n2932 = Equal?(x=w5537, y=w5563) -> (x = y?=w5518:bool)
                      n2933 = Tick Count (ms)() -> (millisecond timer value=w5533:u32)
                      n2934 = Subtract(x=w5533, y=w5562) -> (x-y=w5534:u32)
                      n2935 = Divide(x=w5537, y=w5536) -> (x/y=w5538:sgl)
                      n2936 = local read "Image Update [ms]"() -> (w5530:u32)
                      n2937 = Round Toward +Infinity(x=w5538) -> (ceil(x): smallest int >= x=w5529:sgl)
                      n2938 = Compound Arithmetic op=OR(w5518, w5517, w5516, w5513, w5515) -> (w5514:bool)
                      n2939 = local write "#"(w5529) -> ()
                      n2940 = local read "total y pixels"() -> (w5564:sgl)
                      n2941 = while {
                        tunnel: w5564 -> [w5702]
                        shift-right: [w5703] -> _
                        shift-left: w5495 -> [w5701]
                        tunnel: [w5701] -> w5483
                        tunnel: [w5700] -> w5480
                        i -> [w5700]
                        stop <- w5704 stop-if-true
                        n2942 = Subtract(x=w5701, y=w5702) -> (x-y=w5703:sgl)
                        n2943 = Less?(x=w5701, y=w5702) -> (x < y?=w5704:bool)
                      }
                      n2944 = Index Array(array=w5545, index (col)=w5483) -> (element=w5555:u8[])  [unwired: 1 in]
                      n2945 = Index Array(array=w5484, index (col)=w5483) -> (element=w5485:u8[])  [unwired: 1 in]
                      n2946 = Multiply(x=w5555, y=w5480) -> (x*y=w5554:i32[])
                      n2947 = Greater Or Equal?(x=w5534, y=w5530) -> (x >= y?=w5535:bool)
                      n2948 = Add(x=w5554, y=w5542) -> (x+y=w5552:i32[])
                      n2949 = Multiply(x=w5485, y=w5480) -> (x*y=w5486:i32[])
                      n2950 = Index Array(array=w5543, index (col)=w5483) -> (element=w5546:u8[])  [unwired: 1 in]
                      n2951 = Increment(x=w5480) -> (x+1=w5553:i32)
                      n2952 = Add(x=w5486, y=w5479) -> (x+y=w5488:i32[])
                      n2953 = Multiply(x=w5546, y=w5480) -> (x*y=w5547:i32[])
                      n2954 = Divide(x=w5552, y=w5553) -> (x/y=w5551:dbl[])
                      n2955 = Increment(x=w5480) -> (x+1=w5487:i32)
                      n2956 = Add(x=w5547, y=w5541) -> (x+y=w5549:i32[])
                      n2957 = Increment(x=w5480) -> (x+1=w5548:i32)
                      n2958 = Divide(x=w5488, y=w5487) -> (x/y=w5489:dbl[])
                      n2959 = Replace Array Subset(array=w5545, new element=w5551, index (col)=w5483) -> (w5544:u8[][])  [unwired: 1 in]
                      n2960 = Divide(x=w5549, y=w5548) -> (x/y=w5550:dbl[])
                      n2961 = Replace Array Subset(array=w5484, new element=w5489, index (col)=w5483) -> (w5482:u8[][])  [unwired: 1 in]
                      n2962 = Replace Array Subset(array=w5543, new element=w5550, index (col)=w5483) -> (w5540:u8[][])  [unwired: 1 in]
                      n2963 = case shown="True" w5535 {
                        tunnel: [w5662 w5665] -> w5561
                        tunnel: w5562 -> [w5662 _]
                        tunnel: w5544 -> [_ w5664]
                        tunnel: w5540 -> [_ w5663]
                        frame False {
                        }
                        frame True {
                          n2964 = local write "Image 1"(w5664) -> ()
                          n2965 = local write "Image 2"(w5663) -> ()
                          n2966 = Tick Count (ms)() -> (millisecond timer value=w5665:u32)
                        }
                      }
                    }
                    n2967 = Or(x=w5374, y=w5375) -> (x .or. y?=w5346:bool)
                    n2968 = local write "#"(w5372) -> ()
                    n2969 = Compound Arithmetic op=OR(w5342, w5344, w5343, w5346, w5345) -> (w5327:bool)
                    n2970 = Or(x=w5327, y=w5328) -> (x .or. y?=w5326:bool)
                    n2971 = case shown="True" w5326 {
